vi "VCH VI Tree.vi"   [LabVIEW 2016]
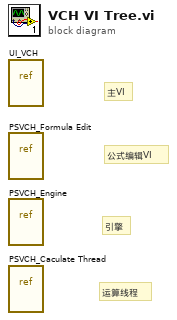
[diagram p0: block diagram]
diagram:
  # "运算线程"
  # "引擎"
  # "公式编辑VI"
  # "主VI"
  n1 = vi-ref "UI_VCH.vi"() -> ()  [unwired: 1 out]
  n2 = vi-ref "PSVCH_Formula Edit.vi"() -> ()  [unwired: 1 out]
  n3 = vi-ref "PSVCH_Engine.vi"() -> ()  [unwired: 1 out]
  n4 = vi-ref "PSVCH_Caculate Thread.vi"() -> ()  [unwired: 1 out]
